vi "Moving Ripple-Initialize.vi"(0 "Params":T2, 5 "Level in":T3, 7 "Sampling rate (Hz)":dbl, 9 "Npts":i32, 11 "error in (no error)":errorcluster) -> (4 "Ripple Data":T1, 15 "error out":errorcluster)   [LabVIEW 2020]
uses:
  Controls/Level XCtl/Level Data.ctl
  Controls/Level XCtl/Level Units.ctl
  Moving Ripple.Params.ctl
  Moving Ripple.Data.ctl
  Utility VIs/Math VIs/LinSpace (x0-dx-npts).vi
  Utility VIs/Math VIs/dB to Linear (1D).vi
  Utility VIs/Math VIs/interp1 (2D).vi
  <vilib>/Analysis/NI_AALBase.lvlib
  Controls/Level XCtl/Level XCtl.xctl
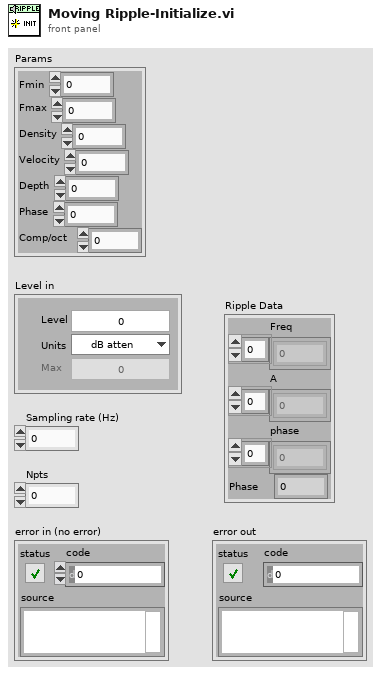
[diagram p1: front panel]
types:
  T1 = typedef "Moving Ripple.Data.ctl" = cluster{"Freq":dbl[], "A":dbl[], "phase":dbl[], "Phase":dbl}
  T2 = typedef "Moving Ripple.Params.ctl" = cluster{"Fmin":dbl, "Fmax":dbl, "Density":dbl, "Velocity":dbl, "Depth":dbl, "Phase":dbl, "Comp/oct":i32}
  T3 = typedef "Level XCtl.xctl/Level Data.ctl" = cluster{"Level":dbl, "Units":T4, "Max":dbl, "Multiplier":dbl, "Cal File":path, "Cal":cluster{"Freq (Hz)":dbl[], "Mag (dB SPL)":dbl[], "Phase (deg)":dbl[]}}
  T4 = typedef "Level Units.ctl" = enum16{"dB atten", "dB SPL", "dB re 1 Vrms", "dB V/Hz½", "mW", "dB HL", "Volts", "dB mW"}
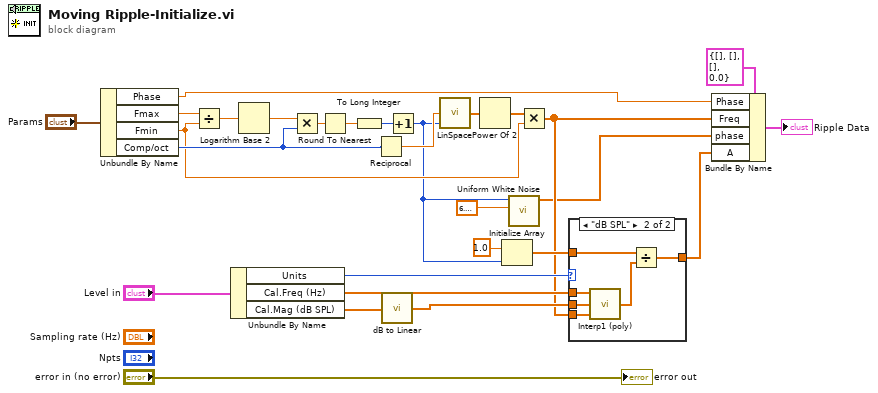
[diagram p0: block diagram]
diagram:
  n1 = Unbundle By Name("Params") -> ("Phase"=w3:dbl, "Fmax"=w27:dbl, "Fmin"=w2:dbl, "Comp/oct"=w12:i32)
  n2 = Divide(x=w27, y=w2) -> (x/y=w26:dbl)
  n3 = Unbundle By Name("Level in") -> ("Units"=w9:T4, "Cal.Freq (Hz)"=w17:dbl[], "Cal.Mag (dB SPL)"=w16:dbl[])
  n4 = Logarithm Base 2(1:w26) -> (0:w25:dbl)
  n5 = Multiply(x=w25, y=w12) -> (x*y=w24:dbl)
  n6 = Round To Nearest(number=w24) -> (nearest integer value=w22:dbl)
  n7 = To Long Integer(number=w22) -> (32bit integer=w23:i32)
  n8 = Reciprocal(x=w12) -> (1/x=w21:dbl)
  n9 = call-poly "dB to Linear.vi"("dB"=w16) -> ("linear"=w15:dbl[])
  n10 = Increment(x=w23) -> (x+1=w1:i32)
  n11 = call-poly "LinSpace.vi"("npts"=w1, "dx"=w21) -> ("Array"=w20:dbl[])  [unwired: 2 in, 1 out]
  n12 = Power Of 2(x=w20) -> (2^x=w19:dbl[])
  n13 = Initialize Array(1.0, w1) -> (w10:dbl[])
  n14 = call <vilib>:"Uniform White Noise.vi"("amplitude"=6.283185307179586, "samples"=w1) -> ("uniform white noise"=w6:dbl[])  [unwired: 8 in, 1 out]
  n15 = Multiply(x=w19, y=w2) -> (x*y=w7:dbl[])
  n16 = case shown="\"dB SPL\"" w9 {
    tunnel: w17 -> [_ w35]
    tunnel: w15 -> [_ w34]
    tunnel: w7 -> [_ w33]
    tunnel: w10 -> [w29 w32]
    tunnel: [w29 w30] -> w5
    frame "dB atten", Default {
    }
    frame "dB SPL" {
      n17 = call-poly "Interp1 (poly).vi"("X"=w35, "Y"=w34, "U"=w33) -> ("V"=w31:dbl[])  [unwired: 2 in]
      n18 = Divide(x=w32, y=w31) -> (x/y=w30:dbl[])
    }
  }
  n19 = Bundle By Name(cluster=T1 {"Freq"=[], "A"=[], "phase"=[], "Phase"=0.0} ("Moving Ripple.Data"), "Phase"=w3, "Freq"=w7, "phase"=w6, "A"=w5) -> (→"Ripple Data":T1)
  "error out" <- "error in (no error)"
